vi "Регистры.vi"(5 "R":bool, 6 "Cluster":T2, 7 "4":T3) -> (0 "4":T1, 1 "3":T1, 2 "2":T1, 3 "1":T1)   [LabVIEW 2017]
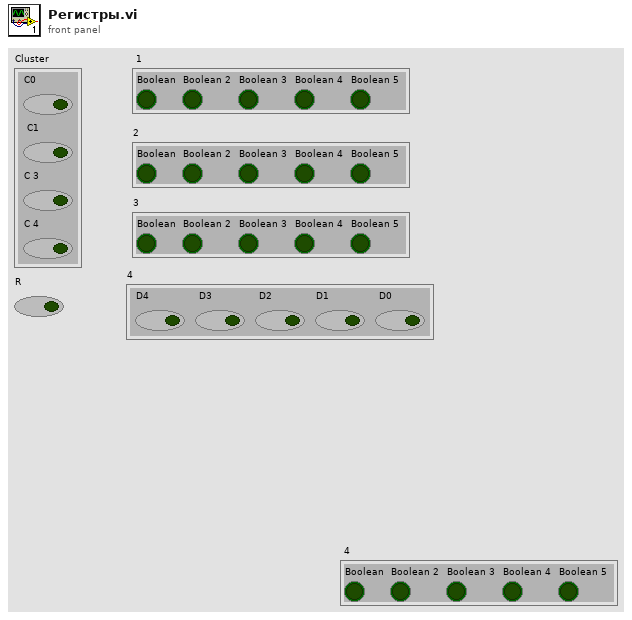
[diagram p1: front panel]
types:
  T1 = cluster{"Boolean":bool, "Boolean 2":bool, "Boolean 3":bool, "Boolean 4":bool, "Boolean 5":bool}
  T2 = cluster{"C0":bool, " C1":bool, "C 3":bool, "C 4":bool}
  T3 = cluster{"D4":bool, " D3":bool, " D2":bool, "D1":bool, " D0":bool}
  T4 = cluster{"q4":bool, "q3":bool, "q2":bool, "q1":bool, "q0":bool}
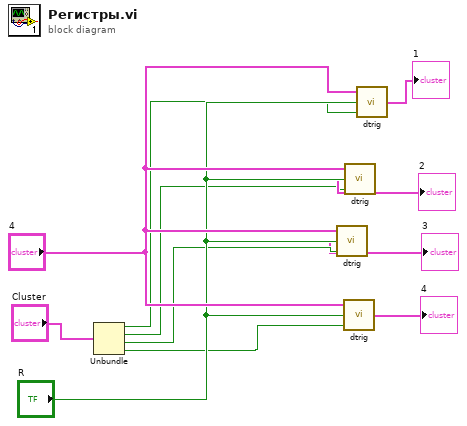
[diagram p0: block diagram]
diagram:
  n1 = Unbundle("Cluster") -> ("C0"=w8:bool, "C1"=w1:bool, "C 3"=w7:bool, "C 4"=w6:bool)
  n2 = call "dtrig.vi"("C"=w7, "RESET"="R", "Cluster"="4") -> ("output cluster"=→"3":T4)
  n3 = call "dtrig.vi"("C"=w6, "RESET"="R", "Cluster"="4") -> ("output cluster"=→"4":T4)
  n4 = call "dtrig.vi"("C"=w1, "RESET"="R", "Cluster"="4") -> ("output cluster"=→"2":T4)
  n5 = call "dtrig.vi"("C"=w8, "RESET"="R", "Cluster"="4") -> ("output cluster"=→"1":T4)
